vi "FreeScale.vi"(6 "LER/NÃO LER":bool, 8 "ESCREVER/NÃO ESCREVER":bool, 9 "milliseconds to wait":u32, 10 "String para Freescale":string, 11 "VISA resource name":refnum<visa-resource-name>) -> (2 "numeros de bits":u32, 3 "string Lido Freescale":string)   [LabVIEW 2019]
uses:
  <vilib>/Instr/_visa.llb/VISA Configure Serial Port (Instr).vi
panel:
  out "error out":errorcluster
  in  "caso programa não\npara, apertar esse\nbotão":bool
  in  "String":string
  in  "data bits (8)":u16=8 min=5 max=8 step=1
  in  "baud rate (9600)":u32=9600
  in  "timeout (10sec)":u32=10000
  # "STRING PARA SER USADA NO CASO DE NÃO TERMOS A PLACA FREESCALE"
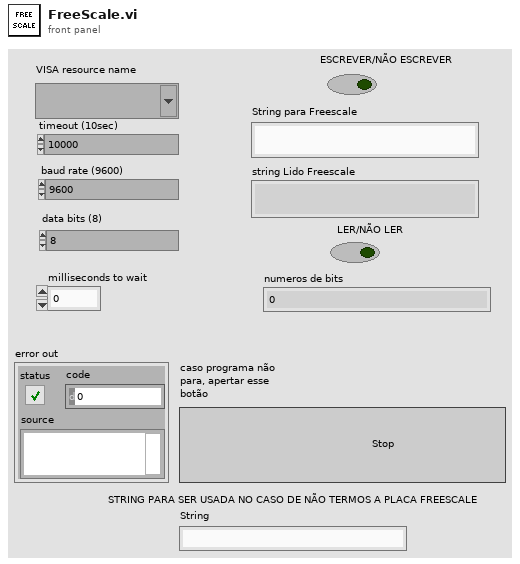
[diagram p1: front panel]
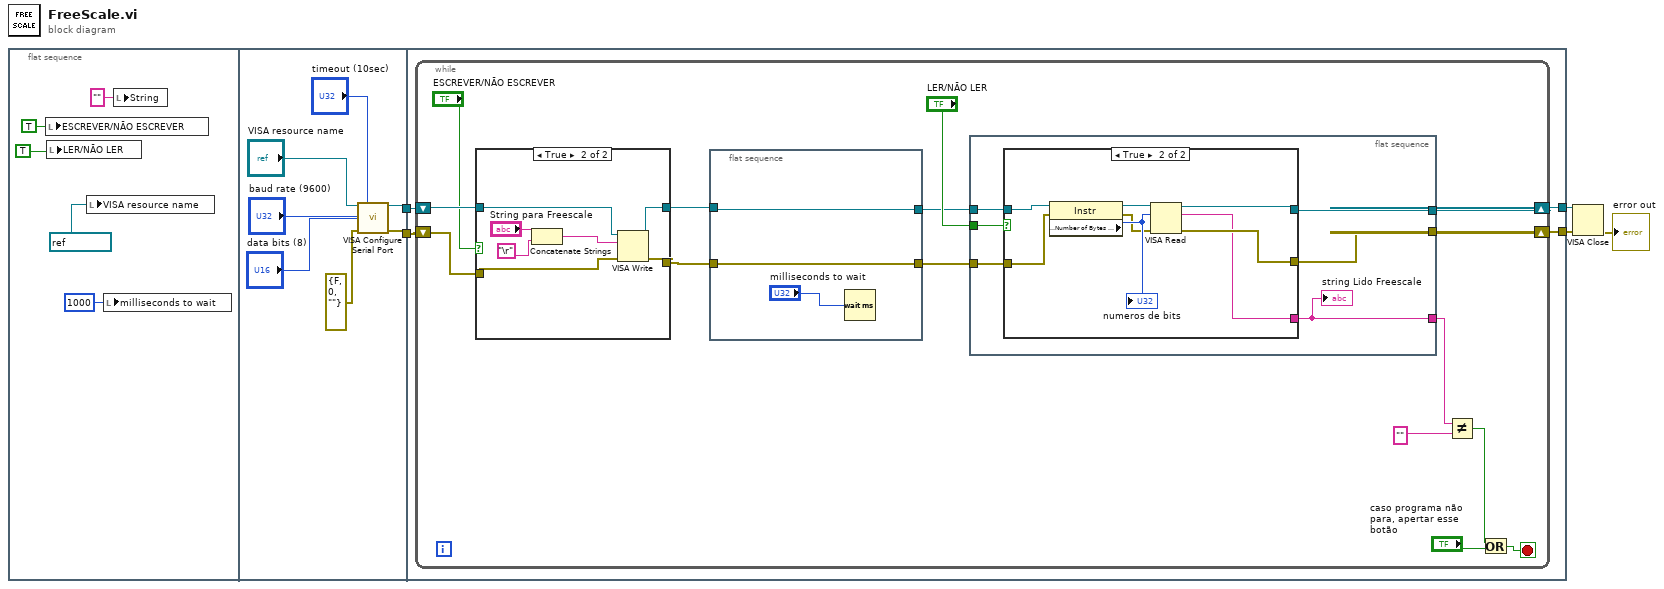
[diagram p0: block diagram]
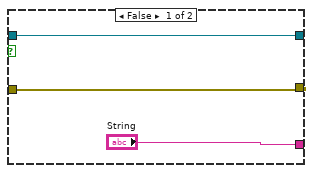
[diagram p2: hidden frame]
diagram:
  n1 = flat-sequence {
    tunnel: [w13] -> w3
    tunnel: [w12] -> w2
    tunnel: [w21] -> w5
    tunnel: [w18] -> w4
    tunnel: w3 -> [w20]
    tunnel: w2 -> [w19]
    frame #0 {
      n2 = local write "ESCREVER/NÃO ESCREVER"(TRUE ("ESCREVER/NÃO ESCREVER")) -> ()
      n3 = local write "LER/NÃO LER"(TRUE ("LER/NÃO LER")) -> ()
      n4 = local write "VISA resource name"(refnum<visa-resource-name> "COM4" ("VISA resource name")) -> ()
      n5 = local write "milliseconds to wait"(u32 1000 ("milliseconds to wait")) -> ()
      n6 = local write "String"("" ("String")) -> ()
    }
    frame #1 {
      n7 = call-poly "VISA Configure Serial Port"("VISA resource name"="VISA resource name", "timeout (10sec)"="timeout (10sec)", "baud rate (9600)"="baud rate (9600)", "data bits (8)"="data bits (8)", "error in (no error)"=errorcluster {"status"=FALSE, "code"=0, "source"=""}) -> ("VISA resource name out"=w13:refnum<visa-resource-name>, "error out"=w12:errorcluster)  [unwired: 9 in]
    }
    frame #2 {
      n8 = while {
        shift-right: [w33] -> w18
        shift-left: w20 -> [w35]
        shift-right: [w36] -> w21
        shift-left: w19 -> [w34]
        stop <- w30 stop-if-true
        n9 = case shown="True" "ESCREVER/NÃO ESCREVER" {
          tunnel: w35 -> [w58 w65]
          tunnel: w34 -> [w57 w64]
          tunnel: [w58 w60] -> w26
          tunnel: [w57 w59] -> w24
          frame False {
          }
          frame True {
            n10 = Concatenate Strings("String para Freescale", "\r" ("string")) -> (w61:string)
            n11 = VISA Write(VISA resource name=w65, write buffer=w61, error in (no error)=w64) -> (VISA resource name out=w60:refnum<visa-resource-name>, error out=w59:errorcluster)  [unwired: 1 out]
          }
        }
        n12 = flat-sequence {
          tunnel: w26 -> [w55]
          tunnel: [w55] -> w25
          tunnel: w24 -> [w54]
          tunnel: [w54] -> w23
          frame #0 {
            n13 = Wait (ms)(milliseconds to wait="milliseconds to wait") -> ()  [unwired: 1 out]
          }
        }
        n14 = flat-sequence {
          tunnel: [w42] -> w36
          tunnel: [w41] -> w33
          tunnel: "LER/NÃO LER" -> [w40]
          tunnel: [w39] -> w27
          tunnel: w25 -> [w38]
          tunnel: w23 -> [w37]
          frame #0 {
            n15 = case shown="True" w40 {
              tunnel: w38 -> [w45 w50]
              tunnel: w37 -> [w44 w49]
              tunnel: [w45 w48] -> w41
              tunnel: [w44 w47] -> w42
              tunnel: ["String" w46] -> w39
              frame False {
              }
              frame True {
                n16 = property class="Instr"(reference=w50, error in=w49) -> (reference out=w52:refnum<visa-resource-name>, error out=w51:errorcluster, "Serial Settings:Number of Bytes at Serial Port"=w53:u32)
                "numeros de bits" <- w53
                n17 = VISA Read(VISA resource name=w52, byte count=w53, error in (no error)=w51) -> (VISA resource name out=w48:refnum<visa-resource-name>, read buffer=w46:string, error out=w47:errorcluster)  [unwired: 1 out]
              }
            }
            "string Lido Freescale" <- w39
          }
        }
        n18 = Not Equal?(x=w27, y="") -> (x != y?=w29:bool)
        n19 = Or(x=w29, y="caso programa não\npara, apertar esse\nbotão") -> (x .or. y?=w30:bool)
      }
    }
  }
  n20 = VISA Close(VISA resource name=w4, error in (no error)=w5) -> (error out=→"error out":errorcluster)
